vi "niDTS GNSS GPS Rx RF Test UTIL Frequency to Channel.vi"(1 "Frequency (Hz) IN":dbl) -> (0 "Channel OUT":T1)   [LabVIEW 2014, in "niDTS GNSS.lvlib"]
uses:
  niDTS GNSS.lvlib
  Includes/niDTS GNSS GPS Rx RF Test INC Channel.ctl
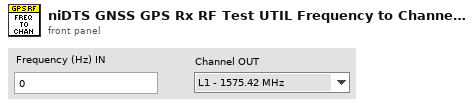
[diagram p1: front panel]
types:
  T1 = typedef "niDTS GNSS.lvlib/niDTS GNSS GPS Rx RF Test INC Channel.ctl" = enum16{"L1 - 1575.42 MHz", "L2 - 1227.60 MHz", "L5 - 1176.45 MHz"}
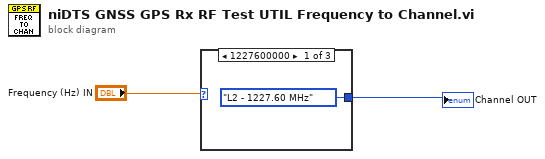
[diagram p0: block diagram]
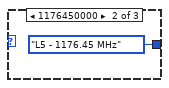
[diagram p2: hidden frame]
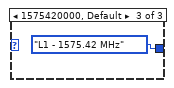
[diagram p3: hidden frame]
diagram:
  n1 = case shown="1227600000" "Frequency (Hz) IN" {
    tunnel: [niDTS_GNSS_GPS_Rx_RF_Test_INC_Channel."L2 - 1227.60 MHz" ("Channel OUT") niDTS_GNSS_GPS_Rx_RF_Test_INC_Channel."L5 - 1176.45 MHz" ("Channel OUT") niDTS_GNSS_GPS_Rx_RF_Test_INC_Channel."L1 - 1575.42 MHz" ("Channel OUT")] -> w1
    frame 1227600000 {
    }
    frame 1176450000 {
    }
    frame 1575420000, Default {
    }
  }
  "Channel OUT" <- w1
